vi "_SizetoRect.vi"(4 "size":cluster{"Width":i32, "Height":i32}) -> (1 "bounds":T1)   [LabVIEW 2012]
doc: "Calculates the bounds for a given rectangle size (width - height)"
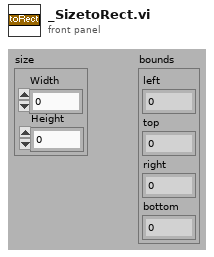
[diagram p1: front panel]
types:
  T1 = cluster{"left":i16, "top":i16, "right":i16, "bottom":i16}
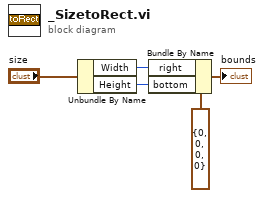
[diagram p0: block diagram]
diagram:
  n1 = Unbundle By Name("size") -> ("Width"=w2:i32, "Height"=w1:i32)
  n2 = Bundle By Name(cluster=T1 {"left"=0, "top"=0, "right"=0, "bottom"=0} ("bounds"), "right"=w2, "bottom"=w1) -> (→"bounds":T1)
